vi "Adv_KillProcessByID.vi"(8 "error in (no error)":errorcluster, 10 "ProcessID":i32, 11 "LightField Automation in":refnum<class "LightField Automation.lvclass">) -> (0 "error out":errorcluster, 3 "LightField Automation out":refnum<class "LightField Automation.lvclass">)   [LabVIEW 2015, in "LightField Automation.lvclass"]
uses:
  LightField Automation.lvclass
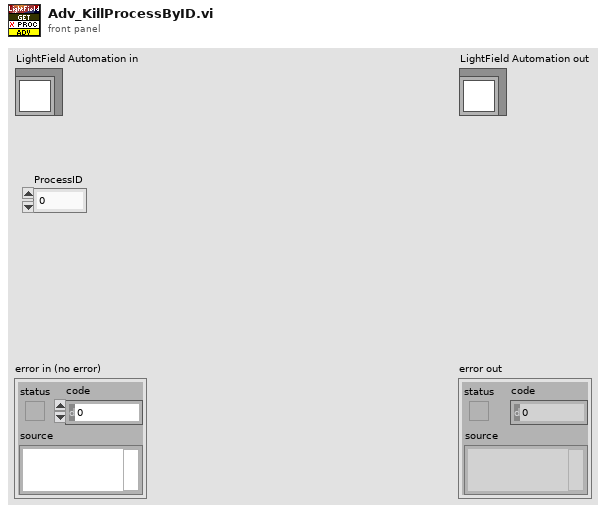
[diagram p1: front panel]
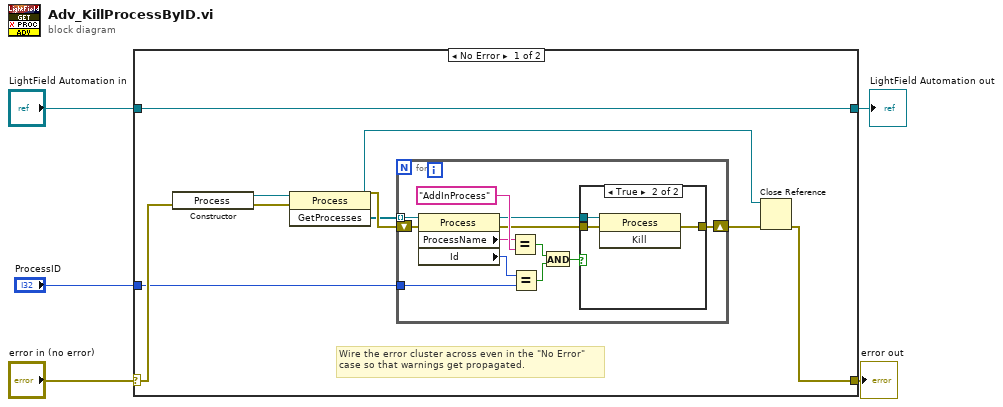
[diagram p0: block diagram]
diagram:
  n1 = case shown="No Error" "error in (no error)" {
    selector: "error in (no error)" -> [w8 w33]
    tunnel: [w6 w33] -> w4
    tunnel: [w15 w32] -> w2
    tunnel: "LightField Automation in" -> [w15 w32]
    tunnel: "ProcessID" -> [w7 _]
    frame No Error {
      # "Wire the error cluster across even in the \"No Error\"\ncase so that warnings get propagated."
      n2 = constructor class="Process"(error in=w8) -> (reference out=w10:refnum<k24>, error out=w9:errorcluster)  [unwired: 2 in, 1 out]
      n3 = invoke class="Process" method="GetProcesses"(reference=w10, error in=w9) -> (reference out=w13:refnum<k24>, error out=w14:errorcluster, "GetProcesses"=w11:refnum<k24>[])  [unwired: 1 in]
      n4 = for {
        tunnel: w11 -> [w26] mode=indexing
        shift-right: [w18] -> w12
        shift-left: w14 -> [w27]
        tunnel: w7 -> [w22]
        n5 = property class="Process"(reference=w26, error in=w27) -> (reference out=w16:refnum<k24>, error out=w17:errorcluster, "ProcessName"=w24:string, "Id"=w23:i32)
        n6 = Equal?(x=w24, y="AddInProcess") -> (x = y?=w20:bool)
        n7 = Equal?(x=w23, y=w22) -> (x = y?=w19:bool)
        n8 = And(x=w20, y=w19) -> (x .and. y?=w21:bool)
        n9 = case shown="True" w21 {
          tunnel: [w28 w29] -> w18
          tunnel: w17 -> [w28 w31]
          tunnel: w16 -> [_ w30]
          frame False {
          }
          frame True {
            n10 = invoke class="Process" method="Kill"(reference=w30, error in=w31) -> (error out=w29:errorcluster)  [unwired: 1 in, 2 out]
          }
        }
      }
      n11 = Close Reference(reference=w13, error in (no error)=w12) -> (error out=w6:errorcluster)
    }
    frame Error {
    }
  }
  "error out" <- w4
  "LightField Automation out" <- w2
